vi "ReadByte.vi"(8 "count":i32, 9 "firstIndex":i32, 10 "HighSpeedEServer":refnum<k24>, 11 "error in (no error)":errorcluster) -> (1 "Value":u8[](array[numeric]), 3 "error out":errorcluster)   [LabVIEW 2020, in "UnderAutomation.Yaskawa.lvlib"]
uses:
  UnderAutomation.Yaskawa.lvlib
  C:/Users/fg/Documents/Yaskawa.vi/LabVIEW_2024/UnderAutomation.Yaskawa/lib/UnderAutomation.Yaskawa.dll
  LabVIEW_2024/UnderAutomation.Yaskawa/lib/UnderAutomation.Yaskawa.dll
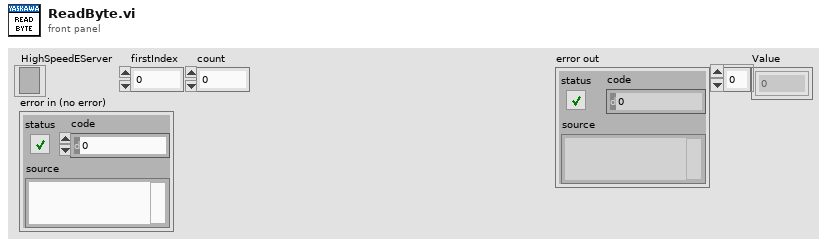
[diagram p1: front panel]
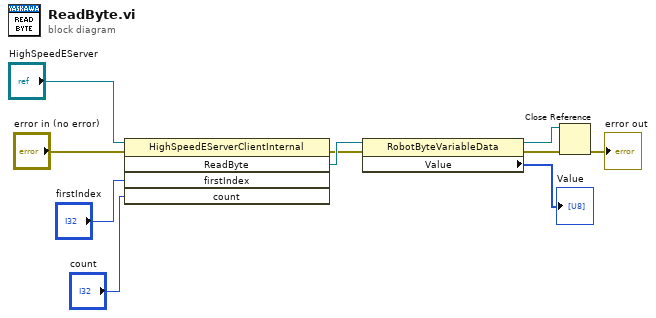
[diagram p0: block diagram]
diagram:
  n1 = invoke class="HighSpeedEServerClientInternal" method="ReadByte"(reference="HighSpeedEServer", error in="error in (no error)", "firstIndex"="firstIndex", "count"="count") -> (error out=w2:errorcluster, "ReadByte"=w6:refnum<k24>)  [unwired: 1 in, 3 out]
  n2 = property class="RobotByteVariableData"(reference=w6, error in=w2) -> (reference out=w3:refnum<k24>, error out=w4:errorcluster, "Value"=→"Value":u8[])
  n3 = Close Reference(reference=w3, error in (no error)=w4) -> (error out=→"error out":errorcluster)
